vi "Interpret Data.vi"   [LabVIEW 2009, in "IDW.lvlib"]
doc: "Changes binary data (bit states '1', '0') into digital waveform data, based on the desired action. This is a low-level VI.\n\nThis VI is polymorphic. It can accept a single byte (<b>U8</b>) or an array of bytes ( <b>[U8]</b> ).\n\nFor a <b>Transmit (Tx)</b> action, bits [1,0] are changed into [Z,0]. For a <b>Receive (Rx)</b> action, bits [1,0] are changed into [H,L].\n\nEach bit of byte is added in the <b>Byte order</b> order, either MSB-first or LSB-first."
uses:
  IDW.lvlib
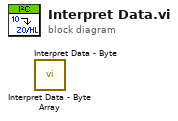
[diagram p0: block diagram]
diagram:
  n1 = call "Interpret Data - Byte Array.vi"() -> ()  [unwired: 10 in, 2 out]
  n2 = call "Interpret Data - Byte.vi"() -> ()  [unwired: 10 in, 2 out]
